vi "_setVIRef.vi"(7 "parentURL":string, 8 "error in (no error)":errorcluster, 10 "Refnum":refnum<vi>, 11 "TagDB in":T1) -> (0 "error out":errorcluster, 2 "URL":string, 3 "TagDB out":T1)   [LabVIEW 2017, in "TagDB RefManager.lvlib"]
uses:
  TagDB RefManager.lvlib
  <userlib>/_NEVSTOP/TagDB/Typedef/TagDB.ctl
  ea13503a-62c4-4b66-bb89-71081f2f96e3.vi
  <userlib>/_NEVSTOP/TagDB/_Support/DataAccess/data-Write.vi
  <userlib>/_NEVSTOP/TagDB/_Support/DataAccess/TagDB Ref to DVR.vi
  <userlib>/_NEVSTOP/TagDB/_Support/DataAccess/_NameCacher.vi
  <userlib>/_NEVSTOP/TagDB/_Support/DataAccess/_datatypeChecker.vi
  <vilib>/Utility/Data Type/Get Type Information.vi
  <userlib>/_NEVSTOP/TagDB/_Support/Error/_[error50000]Invalid DB REF.vi
  <userlib>/_NEVSTOP/TagDB/TagDB.lvlib
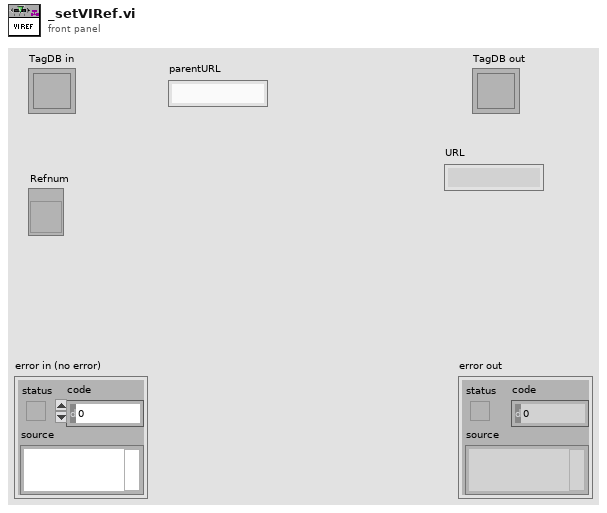
[diagram p1: front panel]
types:
  T1 = typedef "TagDB.lvlib/TagDB.ctl" = refnum<k1>
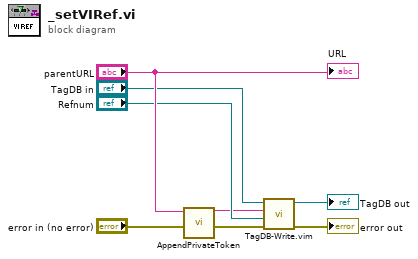
[diagram p0: block diagram]
diagram:
  n1 = call <userlib>:"AppendPrivateToken.vi"("DataURL"="parentURL") -> ("String"=w3:string)  [unwired: 10 in]
  n2 = call "TagDB-Write.vim"("error in (no error)"="error in (no error)", "Value"="Refnum", "tag"=w3, "TagDB"="TagDB in") -> ("error out"=→"error out":errorcluster, "TagDB(dup)"=→"TagDB out":T1)  [unwired: 5 in, 1 out]
  "URL" <- "parentURL"
